vi "CollatePSFCalcs.vi"() -> ()   [LabVIEW 2022 SP3]
uses:
  <vilib>/Analysis/NI_AALBase.lvlib
  <vilib>/Analysis/NI_AALPro.lvlib
  <vilib>/Analysis/5stat.llb/RMS (DBL).vi
panel:
  in  "noise file name":string="40dBNoise_"
  in  "merged file name":string="40dBMerge_"
  in  "dB Noise":dbl=-40.0
  out "Intensity Graph":i16[][](graph)
  out "# rf points per line":u16
  in  "Choose Directory":path
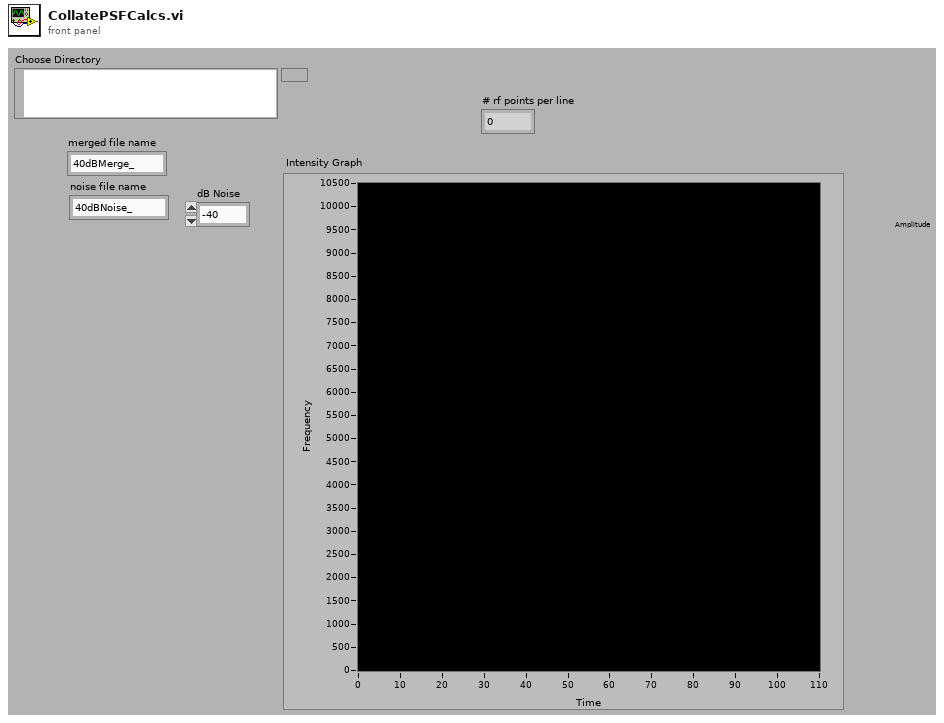
[diagram p1: front panel]
types:
  T1 = cluster{"Digitizer (dB)":sgl, "Gain (dB)":sgl, "Atten (dB)":sgl}
  T2 = typedef "Header.ctl" = cluster{"header info":cluster{"Header":string, "Head length":i16}, "A/D info":cluster{"# rf points per line":u16, "# lines per scan":u16, "sample rate MHz":u16, "# A/D bits":i16, "# bytes per A/D":u16, "TGC Flag":u16, "A/D Type":string}, "Tranducer Info":cluster{"bandwidth":sgl, "center freq":sgl, "start freq":sgl, "ID":i32}, "Scan Info":cluster{"delay":sgl, "pivot distance":sgl, "sector scan angle":sgl, "operator":string, "Scan Mode":string, "location":string}, "Time/Date Info":cluster{"date":string, "time":string}, "RF Info":cluster{"RF file name":string, "RF file att":string, "RF cal file name":string, "RF cal file att":string}, "Patient Info":cluster{"ID":string, "extended ID":string, "age":u16, "sex":string, "previously\nscanned":string, "PSA":sgl, "LOS":u8, "Ethnicty 2":u8, "Race":u8}, "Tissue Type":cluster{"organ":i16, "disease type":i16, "disease location":i16}, "Votage scaling":cluster{"Digitizer (dB)":sgl, "Gain (dB)":sgl, "Atten (dB)":sgl}, "Comment":string, "Misc Info":cluster{"avg num":i16, "c speed":i16, "Div By or SF zones":i16, "XMIT CHS":u8, "RCV CHS":u8}, "Therapy Parameters":cluster{"Theraputic Freq (MHz)":sgl, "Time on (s)":sgl, "Therapy amplitude (mV)":sgl, "Lines Before":u16, "Lines After":u16}, "Scan Settings":cluster{"Energy (uJ or V)":u8, "Damp (Ohm) or Fc":u8, "HP Filt (KHz)":u8, "LP Filt (MHz)":u8, "Gain (db)":u8, "prf (kHz)":sgl, "Distance between\nscan lines (mm)":u16, "Distance between\nscan planes (mm)":u16}, "Compression Parameters":cluster{"F1 (MHz)":sgl, "F2 (MHz)":sgl, "% taper":sgl, "duration":sgl}, "Patient Info Xtra":cluster{"First Name":string, "Last Name":string, "Notes":string}}
  T3 = cluster{"avg num":i16, "c speed":i16, "DivdeBy":i16, "XMIT CHS":u8, "RCV CHS":u8}
  T4 = cluster{"# rf points per line":u16, "# lines per scan":u16, "sample rate MHz":u16, "# A/D bits":i16, "# bytes per A/D":u16, "TGC Flag":u16, "A/D Type":string}
  T5 = cluster{"delay":sgl, "pivot distance":sgl, "sector scan angle":sgl, "operator":string, "Scan Mode":string, "location":string}
  T6 = enum16{"big-endian, network order", "native, host order", "little-endian"}
  T7 = enum16{"open", "replace", "create", "open or create", "replace or create", "replace or create with confirmation"}
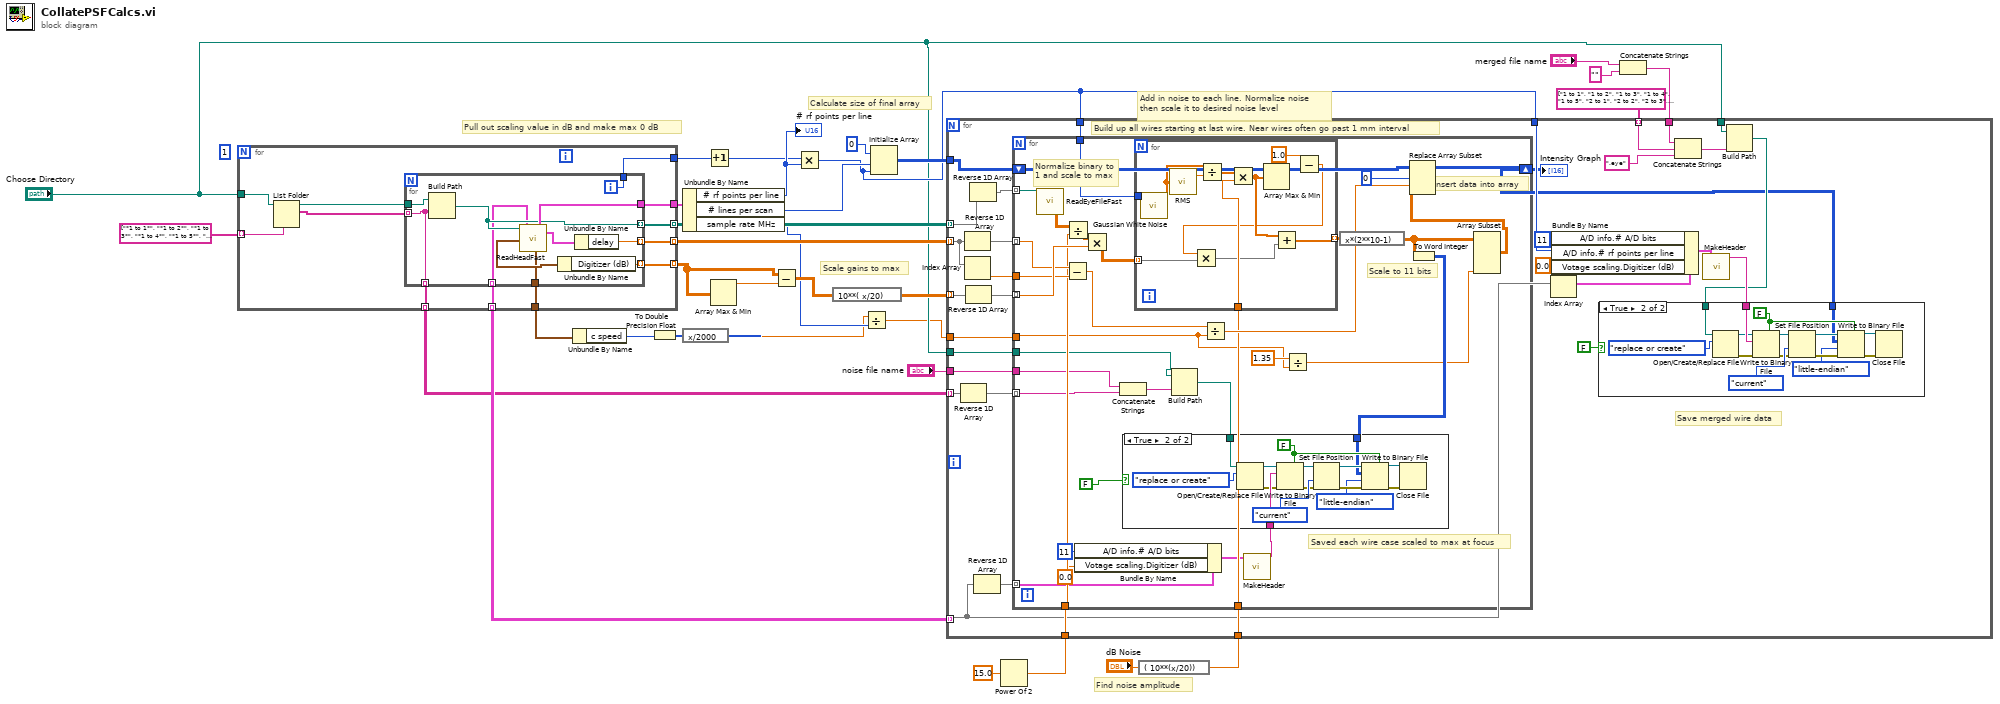
[diagram p0: block diagram]
diagram:
  (unwired) 1
  # "Scale gains to max"
  # "Add in noise to each line. Normalize noise then scale it to desired noise level"
  # "Calculate size of final array"
  # "Pull out scaling value in dB and make max 0 dB"
  # "Find noise amplitude"
  n1 = for {
    tunnel: string[] ["*1 to 1*", "*1 to 2*", "*1 to 3*", "*1 to 4*", "*1 to 5*", "*2 to 1*", "*2 to 2*", "*2 to 3*", "*2 to 4*", "*2 to 5*", "*3 to 1*", "*3 to 2*", "*3 to 3*", "*3 to 4*", "*3 to 5*", "*4 to 1*", "*4 to 2*", "*4 to 3*", "*4 to 4*", "*4 to 5*", "*5 to 1*", "*5 to 2*", "*5 to 3*", "*5 to 4*", "*5 to 5*"] ("Array 2") -> [w45] mode=indexing
    tunnel: "Choose Directory" -> [w44]
    tunnel: [w41] -> w30 mode=indexing
    tunnel: [w40] -> w32
    tunnel: [w39] -> w6
    tunnel: [w38] -> w24 mode=indexing
    tunnel: [w37] -> w23
    tunnel: [w36] -> w10 mode=indexing
    tunnel: [w35] -> w9 mode=indexing
    tunnel: [w34] -> w8 mode=indexing
    n2 = List Folder(path=w44, pattern=w45) -> (path out=w43:path, filenames=w42:string[])  [unwired: 1 in, 3 out]
    n3 = for {
      tunnel: w43 -> [w56]
      tunnel: w42 -> [w46] mode=indexing
      tunnel: [w54] -> w41 mode=indexing
      tunnel: [w53] -> w40
      tunnel: [w52] -> w39
      tunnel: [w51] -> w38 mode=indexing
      tunnel: [w50] -> w37
      tunnel: [w48] -> w36 mode=indexing
      tunnel: [w47] -> w35 mode=indexing
      tunnel: [w46] -> w34 mode=indexing
      i -> [w52]
      n4 = Build Path(base path=w56, name or relative path=w46) -> (appended path=w51:path)
      n5 = call "ReadHeadFast.vi"("new file path"=w51) -> ("Votage scaling"=w55:T1, "Header In"=w47:T2, "Misc Items"=w50:T3, "A/D info"=w53:T4, "Scan Info"=w49:T5)  [unwired: 2 in, 12 out]
      n6 = Unbundle By Name(w55) -> ("Digitizer (dB)"=w54:sgl)
      n7 = Unbundle By Name(w49) -> ("delay"=w48:sgl)
    }
  }
  n8 = Unbundle By Name(w23) -> ("c speed"=w16:i16)
  n9 = To Double Precision Float(number=w16) -> (double precision float=w15:dbl)
  n10 = Unbundle By Name(w32) -> ("# rf points per line"=w31:u16, "# lines per scan"=w28:u16, "sample rate MHz"=w3:u16)
  "# rf points per line" <- w31
  n11 = expression code="x/2000"(w15) -> (w2:dbl)
  n12 = Increment(x=w6) -> (x+1=w5:i32)
  n13 = Array Max & Min(array=w30) -> (max value=w29:sgl)  [unwired: 3 out]
  n14 = Subtract(x=w30, y=w29) -> (x-y=w26:sgl[][])
  n15 = Multiply(x=w5, y=w31) -> (x*y=w13:i32)
  n16 = expression code="10**( x/20)"(w26) -> (w22:sgl[][])
  n17 = Divide(x=w2, y=w3) -> (x/y=w1:dbl)
  n18 = Initialize Array(i16 0 ("element"), w28, w13) -> (w25:i16[][])
  n19 = Power Of 2(x=15.0) -> (2^x=w12:dbl)
  n20 = expression code="( 10**(x/20))"("dB Noise") -> (w11:dbl)
  n21 = Concatenate Strings("merged file name", "" ("string")) -> (w18:string)
  n22 = for {
    tunnel: w22 -> [w64] mode=indexing
    tunnel: w25 -> [w88]
    tunnel: w24 -> [w66] mode=indexing
    tunnel: w1 -> [w75]
    tunnel: w10 -> [w65] mode=indexing
    tunnel: w9 -> [w62] mode=indexing
    tunnel: w13 -> [w85]
    tunnel: w13 -> [w82]
    tunnel: w18 -> [w81]
    tunnel: string[] ["1 to 1", "1 to 2", "1 to 3", "1 to 4", "1 to 5", "2 to 1", "2 to 2", "2 to 3", "2 to 4", "2 to 5", "3 to 1", "3 to 2", "3 to 3", "3 to 4", "3 to 5", "4 to 1", "4 to 2", "4 to 3", "4 to 4", "4 to 5", "5 to 1", "5 to 2", "5 to 3", "5 to 4", "5 to 5"] ("Array") -> [w80] mode=indexing
    tunnel: "Choose Directory" -> [w77]
    tunnel: w11 -> [w74]
    tunnel: w12 -> [w71]
    tunnel: w8 -> [w63] mode=indexing
    tunnel: "Choose Directory" -> [w69]
    tunnel: "noise file name" -> [w67]
    # "Build up all wires starting at last wire. Near wires often go past 1 mm interval"
    # "Save merged wire data"
    n23 = Reverse 1D Array(array=w63) -> (reversed array=w58:string[])
    n24 = Reverse 1D Array(array=w65) -> (reversed array=w60:sgl[])
    n25 = Index Array(array=w65) -> (element=w87:sgl)  [unwired: 1 in]
    n26 = Reverse 1D Array(array=w64) -> (reversed array=w59:sgl[])
    n27 = Reverse 1D Array(array=w66) -> (reversed array=w61:path[])
    n28 = Reverse 1D Array(array=w62) -> (reversed array=w57:T2[])
    n29 = for {
      tunnel: w59 -> [w133] mode=indexing
      tunnel: w61 -> [w136] mode=indexing
      shift-right: [w111] -> w68
      shift-left: w88 -> [w135]
      tunnel: w60 -> [w131] mode=indexing
      tunnel: w87 -> [w130]
      tunnel: w82 -> [w128]
      tunnel: w75 -> [w106]
      tunnel: w74 -> [w127]
      tunnel: w71 -> [w124]
      tunnel: w57 -> [w118] mode=indexing
      tunnel: w58 -> [w115] mode=indexing
      tunnel: w69 -> [w113]
      tunnel: w67 -> [w110]
      # "Normalize binary to 1 and scale to max"
      # "Insert data into array"
      # "Scale to 11 bits"
      # "Saved each wire case scaled to max at focus"
      n30 = call "ReadEyeFileFast.vi"("new file path"=w136) -> ("2-D data array"=w126:sgl[][])  [unwired: 1 in, 17 out]
      n31 = Subtract(x=w131, y=w130) -> (x-y=w129:sgl)
      n32 = Divide(x=w126, y=w124) -> (x/y=w125:dbl[][])
      n33 = Bundle By Name(cluster=w118, "A/D info.# A/D bits"=i16 11, "Votage scaling.Digitizer (dB)"=sgl 0.0) -> (w122:T2)
      n34 = Multiply(x=w125, y=w133) -> (x*y=w104:dbl[][])
      n35 = Concatenate Strings(w110, w115) -> (w116:string)
      n36 = for {
        tunnel: [w163] -> w112 mode=indexing
        tunnel: w128 -> [w162]
        tunnel: w127 -> [w157]
        tunnel: w104 -> [w154] mode=indexing
        n37 = call <vilib>:"Gaussian White Noise.vi"("samples"=w162) -> ("Gaussian noise pattern"=w161:dbl[])  [unwired: 9 in, 1 out]
        n38 = call-poly <vilib>:"RMS.vi"("X"=w161) -> ("rms value"=w160:dbl)  [unwired: 1 out]
        n39 = Divide(x=w161, y=w160) -> (x/y=w159:dbl[])
        n40 = Multiply(x=w159, y=w157) -> (x*y=w158:dbl[])
        n41 = Array Max & Min(array=w158) -> (max value=w156:dbl)  [unwired: 3 out]
        n42 = Subtract(x=1.0, y=w156) -> (x-y=w153:dbl)
        n43 = Multiply(x=w153, y=w154) -> (x*y=w152:dbl[])
        n44 = Add(x=w158, y=w152) -> (x+y=w163:dbl[])
      }
      n45 = Build Path(base path=w113, name or relative path=w116) -> (appended path=w114:path)
      n46 = Divide(x=w129, y=w106) -> (x/y=w134:dbl)
      n47 = call "MakeHeader.vi"("Header In"=w122) -> ("Header String"=w119:string)  [unwired: 6 out]
      n48 = Divide(x=1.35, y=w106) -> (x/y=w105:dbl)
      n49 = expression code="x*(2**10-1)"(w112) -> (w108:dbl[][])
      n50 = To Word Integer(number=w108) -> (16bit integer=w117:i16[][])
      n51 = case shown="True" FALSE {
        tunnel: w119 -> [_ w151]
        tunnel: w117 -> [_ w138]
        tunnel: w114 -> [_ w137]
        frame False {
        }
        frame True {
          w140 = FALSE ("prepend array or string size? (T)")
          n52 = Open/Create/Replace File(file path (use dialog)=w137, operation (0:open)=T7."replace or create") -> (refnum out=w144:refnum<file>, error out=w143:errorcluster)  [unwired: 1 in, 4 out]
          n53 = Write to Binary File(file (use dialog)=w144, data=w151, error in=w143, 5:w140) -> (refnum out=w146:refnum<file>, error out=w145:errorcluster)  [unwired: 3 out]
          n54 = Set File Position(refnum=w146, from (0:start)=enum16{"start", "end", "current"}."current" ("pos mode (0:2)"), error in=w145) -> (refnum out=w142:refnum<file>, error out=w141:errorcluster)  [unwired: 1 out]
          n55 = Write to Binary File(file (use dialog)=w142, data=w138, error in=w141, 5:w140, 9:T6."little-endian" ("byte order (0:big-endian, network order)")) -> (refnum out=w148:refnum<file>, error out=w149:errorcluster)  [unwired: 2 out]
          n56 = Close File(refnum=w148, error in=w149) -> ()  [unwired: 2 out]
        }
      }
      n57 = Array Subset(array=w108, length (col)=w105) -> (w109:dbl[][])  [unwired: 3 in]
      n58 = Replace Array Subset(array=w135, new element=w109, index (row)=0 ("disabled index (row)"), index (col)=w134) -> (w111:i16[][])
    }
    "Intensity Graph" <- w68
    n59 = Index Array(array=w62) -> (element=w70:T2)  [unwired: 1 in]
    n60 = Bundle By Name(cluster=w70, "A/D info.# A/D bits"=i16 11, "A/D info.# rf points per line"=w85, "Votage scaling.Digitizer (dB)"=sgl 0.0) -> (w83:T2)
    n61 = Concatenate Strings(w81, w80, ".eye" ("string")) -> (w78:string)
    n62 = call "MakeHeader.vi"("Header In"=w83) -> ("Header String"=w86:string)  [unwired: 6 out]
    n63 = Build Path(base path=w77, name or relative path=w78) -> (appended path=w76:path)
    n64 = case shown="True" FALSE {
      tunnel: w86 -> [_ w103]
      tunnel: w68 -> [_ w90]
      tunnel: w76 -> [_ w89]
      frame False {
      }
      frame True {
        w92 = FALSE ("prepend array or string size? (T)")
        n65 = Open/Create/Replace File(file path (use dialog)=w89, operation (0:open)=T7."replace or create") -> (refnum out=w96:refnum<file>, error out=w95:errorcluster)  [unwired: 1 in, 4 out]
        n66 = Write to Binary File(file (use dialog)=w96, data=w103, error in=w95, 5:w92) -> (refnum out=w98:refnum<file>, error out=w97:errorcluster)  [unwired: 3 out]
        n67 = Set File Position(refnum=w98, from (0:start)=enum16{"start", "end", "current"}."current" ("pos mode (0:2)"), error in=w97) -> (refnum out=w94:refnum<file>, error out=w93:errorcluster)  [unwired: 1 out]
        n68 = Write to Binary File(file (use dialog)=w94, data=w90, error in=w93, 5:w92, 9:T6."little-endian" ("byte order (0:big-endian, network order)")) -> (refnum out=w100:refnum<file>, error out=w101:errorcluster)  [unwired: 2 out]
        n69 = Close File(refnum=w100, error in=w101) -> ()  [unwired: 2 out]
      }
    }
  }
